vi "Cargo Intake.vi"   [LabVIEW 2018]
uses:
  <vilib>/Rock Robotics/WPI/Solenoid/WPI_SolenoidChannel.ctl
  <vilib>/Rock Robotics/WPI/ThirdParty/Phoenix-LabVIEW/Motor Controller/Controls/CTRE_Phoenix_MotorControl_ControlMode.ctl
  <vilib>/Rock Robotics/WPI/Solenoid/WPI_SolenoidValue.ctl
  Cargo Intake Global.vi
  <vilib>/Rock Robotics/WPI/Solenoid/WPI_SolenoidOpenSingle.vi
  Sensors/Sensors Global.vi
  Times/Times Global.vi
  <vilib>/Rock Robotics/WPI/Solenoid/WPI_SolenoidSetEnum.vi
types:
  T1 = typedef "WPI_SolenoidChannel.ctl" = enum8{"Solenoid 0", "Solenoid 1", "Solenoid 2", "Solenoid 3", "Solenoid 4", "Solenoid 5", "Solenoid 6", "Solenoid 7", "Invalid"}
  T2 = enum16{"Full Manual Control", "Manual Control", "Automated Control"}
  T3 = typedef "WPI_SolenoidValue.ctl" = enum16{"Off", "On", "Forward", "Reverse"}
  T4 = typedef "WPI_SolenoidDevRef.ctl" = cluster{"DevStatus":errorcluster, "Pneumatics Control Module":u8, "Forward Solenoid Channel":T1, "Reverse Solenoid Channel":T1}
  T5 = typedef "WPI_MotorControlDeviceRef.ctl" = cluster{"DeviceStatus":errorcluster, "Type":T6, "PWM":cluster{"PWM Channel":T7, "DeadBand":T8}, "CAN":cluster{"Device Number":u8, "SetOutput VI Ref":variant, "GetOutput VI Ref":variant, "Enable VI Ref":variant, "Disable VI Ref":variant, "Data":variant}, "Invert":bool, "DIO PWM":cluster{"PWM \"Enable\" Channel":T7, "DIOChannel":T9, "PWM Rate":dbl}}
  T6 = typedef "WPI_MotorControlType.ctl" = enum16{"PWM", "CAN", "DIO PWM"}
  T7 = typedef "FPGA_DIOPWMChannel.ctl" = enum8{"PWM 0", "PWM 1", "PWM 2", "PWM 3", "PWM 4", "PWM 5", "PWM 6", "PWM 7", "PWM 8", "PWM 9", "PWM MXP 0", "PWM MXP 1", "PWM MXP 2", "PWM MXP 3", "PWM MXP 4", "PWM MXP 5", "PWM MXP 6", "PWM MXP 7", "PWM MXP 8", "PWM MXP 9", "Invalid"}
  T8 = typedef "WPI_PWMDeadband.ctl" = cluster{"Name":string, "maxPositivePwm":i32, "minPositivePwm":i32, "centerPwm":i32, "maxNegativePwm":i32, "minNegativePwm":i32, "angularRange":u16}
  T9 = typedef "FPGA_DIOChannel.ctl" = enum8{"DIO 0", "DIO 1", "DIO 2", "DIO 3", "DIO 4", "DIO 5", "DIO 6", "DIO 7", "DIO 8", "DIO 9", "DIO MXP 0", "DIO MXP 1", "DIO MXP 2", "DIO MXP 3", "DIO MXP 4", "DIO MXP 5", "DIO MXP 6", "DIO MXP 7", "DIO MXP 8", "DIO MXP 9", "DIO MXP 10", "DIO MXP 11", "DIO MXP 12", "DIO MXP 13", "DIO MXP 14", "DIO MXP 15", "SPI Port CS1", "SPI Port CS2", "SPI Port CS3", "SPI Port MISO", "SPI Port MOSI", "Invalid"}
  T10 = typedef "CTRE_Phoenix_MotorControl_ControlMode.ctl" = u16
  T11 = typedef "Control 1.ctl" = dbl
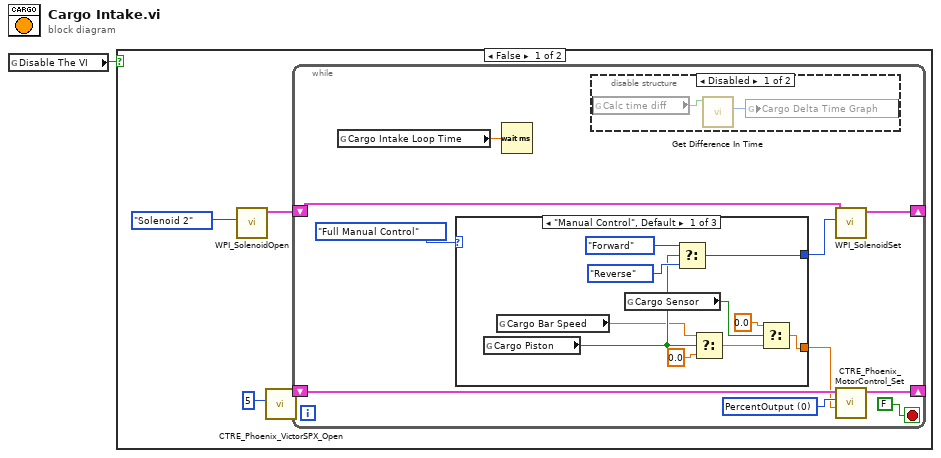
[diagram p0: block diagram]
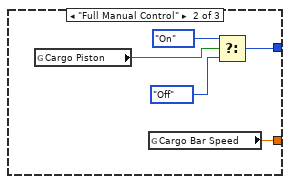
[diagram p3: hidden frame]
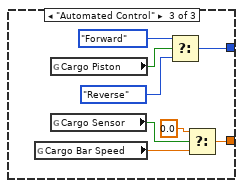
[diagram p4: hidden frame]
diagram:
  n1 = global read "Cargo Intake Global.vi" "Disable The VI"() -> (w1:bool)
  n2 = case shown="False" w1 {
    frame False {
      n3 = call-poly <vilib>:"WPI_SolenoidOpen.vi"("Solenoid Channel"=WPI_SolenoidChannel."Solenoid 2") -> ("SolenoidDevRef"=w2:T4)  [unwired: 9 in, 1 out]
      n4 = call <vilib>:"CTRE_Phoenix_VictorSPX_Open.vi"("Device Number"=u8 5) -> ("CAN Talon SRX Ref"=w4:T5)  [unwired: 9 in, 1 out]
      n5 = while {
        shift-right: [w12] -> _
        shift-left: w4 -> [w10]
        shift-right: [w8] -> _
        shift-left: w2 -> [w6]
        stop <- FALSE stop-if-true
        w11 = T10 0 items=["PercentOutput"=0, "Position"=1, "Velocity"=2, "Current"=3, "Follower"=5, "MotionProfile"=6, "MotionMagic"=7, "MotionProfileArc"=10, "Disabled"=15] ("Control Mode")
        n6 = global read "Times Global.vi" "Cargo Intake Loop Time"() -> (w15:T11)
        n7 = case shown="\"Manual Control\", Default" T2."Full Manual Control" ("Cargo Intake Mode") {
          tunnel: [w25 w32 w40] -> w9
          tunnel: [w21 w29 w35] -> w7
          frame "Manual Control", Default {
            n8 = global read "Cargo Intake Global.vi" "Cargo Piston"() -> (w19:bool)
            n9 = global read "Cargo Intake Global.vi" "Cargo Bar Speed"() -> (w18:dbl)
            n10 = global read "Sensors Global.vi" "Cargo Sensor"() -> (w20:bool)
            n11 = Select(t=WPI_SolenoidValue."Forward" ("Value"), s=w19, f=WPI_SolenoidValue."Reverse" ("Value")) -> (s? t:f=w21:T3)
            n12 = Select(t=w18, s=w19, f=0.0 ("t")) -> (s? t:f=w27:dbl)
            n13 = Select(t=0.0, s=w20, f=w27) -> (s? t:f=w25:dbl)
          }
          frame "Full Manual Control" {
            n14 = global read "Cargo Intake Global.vi" "Cargo Piston"() -> (w28:bool)
            n15 = global read "Cargo Intake Global.vi" "Cargo Bar Speed"() -> (w32:dbl)
            n16 = Select(t=WPI_SolenoidValue."On" ("Value"), s=w28, f=WPI_SolenoidValue."Off" ("Value")) -> (s? t:f=w29:T3)
          }
          frame "Automated Control" {
            n17 = global read "Cargo Intake Global.vi" "Cargo Bar Speed"() -> (w38:dbl)
            n18 = global read "Cargo Intake Global.vi" "Cargo Piston"() -> (w34:bool)
            n19 = global read "Sensors Global.vi" "Cargo Sensor"() -> (w33:bool)
            n20 = Select(t=WPI_SolenoidValue."Forward" ("Value"), s=w34, f=WPI_SolenoidValue."Reverse" ("Value")) -> (s? t:f=w35:T3)
            n21 = Select(t=0.0, s=w33, f=w38) -> (s? t:f=w40:dbl)
          }
        }
        n22 = Wait (ms)(milliseconds to wait=w15) -> ()  [unwired: 1 out]
        n23 = disable-structure shown="Disabled" {
          frame Disabled {
            n24 = global read "Cargo Intake Global.vi" "Calc time diff"() -> (w17:bool)
            n25 = call "Get Difference In Time.vi"("Calculate Time Difference"=w17) -> ("Delta Time over Time"=w16:u32)  [unwired: 9 in, 1 out]
            n26 = global write "Times Global.vi" "Cargo Delta Time Graph"(w16) -> ()
          }
          frame Enabled {
          }
        }
        n27 = call-poly <vilib>:"WPI_SolenoidSet.vi"("Value"=w7, "SolenoidDevRef"=w6) -> ("SolenoidDevRef"=w8:T4)  [unwired: 8 in, 1 out]
        n28 = call <vilib>:"CTRE_Phoenix_MotorControl_Set.vi"("Output"=w9, "Control Mode"=w11, "PhoenixMotorControlDevRef"=w10) -> ("PhoenixMotorControlDevRef"=w12:T5)  [unwired: 7 in, 1 out]
      }
    }
    frame True {
    }
  }
